vi "setflightmode.vi"(0 "stabilise":bool, 1 "althold":bool, 2 "poshold":bool, 3 "loiter":bool, 4 "rtl":bool, 5 "land":bool, 6 "LabVIEW Web Service Request":refnum<class "Web Request.lvclass">, 7 "autotune":bool) -> ()   [LabVIEW 2014]
uses:
  <vilib>/wsapi/Web Request.lvclass
  DronePi Global Variables.vi
panel:
  # "Each additional control wired to the connector pane will be available as an input in the URL. To include an indicator in terminal-mode output (the default setting), it must also be wired to the connector pane."
  # "Use the Web Service Request input terminal to call the VIs on the Web Services palette. Do not remove it from the connector pane unless you don't need access to the palette."
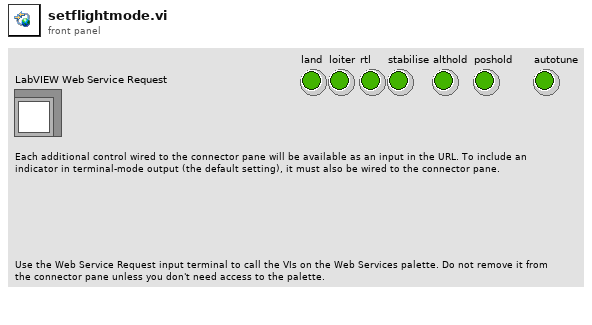
[diagram p1: front panel]
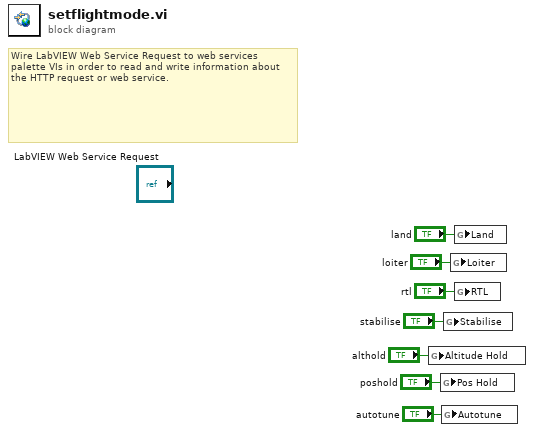
[diagram p0: block diagram]
diagram:
  # "Wire LabVIEW Web Service Request to web services palette VIs in order to read and write information about the HTTP request or web service."
  n1 = global write "DronePi Global Variables.vi" "Altitude Hold"("althold") -> ()
  n2 = global write "DronePi Global Variables.vi" "Pos Hold"("poshold") -> ()
  n3 = global write "DronePi Global Variables.vi" "Autotune"("autotune") -> ()
  n4 = global write "DronePi Global Variables.vi" "Stabilise"("stabilise") -> ()
  n5 = global write "DronePi Global Variables.vi" "Loiter"("loiter") -> ()
  n6 = global write "DronePi Global Variables.vi" "Land"("land") -> ()
  n7 = global write "DronePi Global Variables.vi" "RTL"("rtl") -> ()
